vi "BuildTerminalLabelName.vi"(1 "CloneID":i32, 2 "CRef Type":T1, 3 "Bounds":T2, 4 "VI Name":string) -> (0 "Label Name":string)   [LabVIEW 2012]
uses:
  <vilib>/Utility/miscctls.llb/LVRectTypeDef.ctl
  CRef/Core/Master Types.ctl
  CRef/CRef.lvlib
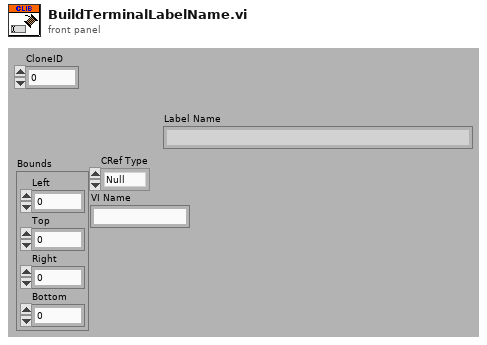
[diagram p1: front panel]
types:
  T1 = typedef "CRef.lvlib/Master Types.ctl" = enum8{"Null", "Boolean", "U8", "I8", "U16", "I16", "U32", "I32", "U64", "I64", "Single", "Double", "Extended", "CSG", "CDB", "CXT", "Boolean(Def)", "U8(Def)", "I8(Def)", "U16(Def)", "I16(Def)", "U32(Def)", "I32(Def)", "Reserved Def", "Reserved Def1", "Single(Def)", "Double(Def)", "Reserved Def2", "Reserved Def3", "Reserved Def4", "Reserved Def5", "Unsigned(Def)", "Signed(Def)", "Real(Def)", "Reserved Def6", "Numeric(Def)", "String"}
  T2 = typedef "LVRectTypeDef.ctl" = cluster{"Left":i16, "Top":i16, "Right":i16, "Bottom":i16}
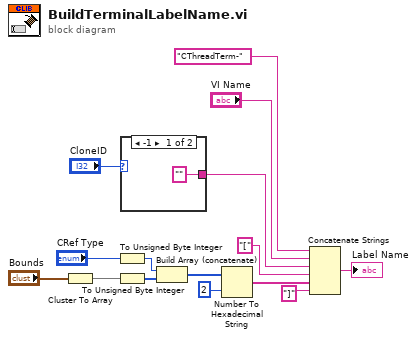
[diagram p0: block diagram]
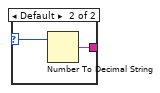
[diagram p2: hidden frame]
diagram:
  n1 = Cluster To Array(cluster="Bounds") -> (array=w15:i16[])
  n2 = To Unsigned Byte Integer(number="CRef Type") -> (unsigned 8bit integer=w13:u8)
  n3 = To Unsigned Byte Integer(number=w15) -> (unsigned 8bit integer=w14:u8[])
  n4 = case shown="-1" "CloneID" {
    selector: "CloneID" -> [_ w17]
    tunnel: ["" w18] -> w2
    frame -1 {
    }
    frame Default {
      n5 = Number To Decimal String(number=w17) -> (decimal integer string=w18:string)  [unwired: 1 in]
    }
  }
  n6 = Build Array (concatenate)(w13, w14) -> (w8:u8[])
  n7 = Number To Hexadecimal String(1:i16 2 ("width (-)"), 2:w8) -> (0:w7:string[])
  n8 = Concatenate Strings("CThreadTerm-", "VI Name", w2, "[" ("string"), w7, "]" ("string")) -> (→"Label Name":string)
